vi "数据库读取.vi"(4 "error in (no error)":errorcluster caption="错误输入（无错误）", 6 "Container State":T6 caption="容器状态", 7 "Display State In":T1={"扫描参数"={"+ V"=0.0, "+ Δ V"=0.0, "+ limit I"=0.01, "- V"=0.0, "- Δ V"=0.0, "- limit I"=0.01, "ΔT"=0.0, "NPLC"=0.001}, "保持时间"={"+ V"=0.0, "+ limit I"=0.01, "T"=0.0, "ΔT"=0.0, "NPLC"=0.001}, "功能选择"=enum."扫描", "强制时序"=FALSE, "数据库引用"=refnum} caption="显示状态输入" {"保持时间"."ΔT" format="%#_6ps"; "保持时间"."T" format="%#_6ps"; "保持时间"."NPLC" min=0.001 max=25.0 step=0.001; "保持时间"."+ limit I" min=1e-08 max=3.0 format="%#_6pA"; "保持时间"."+ V" min=-40.0 max=40.0 format="%#_6pV"; "扫描参数"."NPLC" min=0.001 max=25.0 step=0.001; "扫描参数"."- Δ V" min=0.0 max=1.0 format="%#_6pV"; "扫描参数"."+ Δ V" min=0.0 max=1.0 format="%#_6pV"; "扫描参数"."- V" min=-40.0 max=40.0 format="%#_6pV"; "扫描参数"."- limit I" min=1e-08 max=3.0 format="%#_6pA"; "扫描参数"."ΔT" format="%#_6ps"; "扫描参数"."+ limit I" min=1e-08 max=3.0 format="%#_6pA"; "扫描参数"."+ V" min=-40.0 max=40.0 format="%#_6pV"}) -> (0 "error out":errorcluster caption="错误输出", 2 "Value":T5 caption="值", 3 "Display State Out":T1={"扫描参数"={"+ V"=0.0, "+ Δ V"=0.0, "+ limit I"=0.01, "- V"=0.0, "- Δ V"=0.0, "- limit I"=0.01, "ΔT"=0.0, "NPLC"=0.001}, "保持时间"={"+ V"=0.0, "+ limit I"=0.01, "T"=0.0, "ΔT"=0.0, "NPLC"=0.001}, "功能选择"=enum."扫描", "强制时序"=FALSE, "数据库引用"=refnum} caption="显示状态输出" {"保持时间"."ΔT" format="%#_6ps"; "保持时间"."T" format="%#_6ps"; "保持时间"."NPLC" min=0.001 max=25.0 step=0.001; "保持时间"."+ limit I" min=1e-08 max=3.0 format="%#_6pA"; "保持时间"."+ V" min=-40.0 max=40.0 format="%#_6pV"; "扫描参数"."NPLC" min=0.001 max=25.0 step=0.001; "扫描参数"."- Δ V" min=0.0 max=1.0 format="%#_6pV"; "扫描参数"."+ Δ V" min=0.0 max=1.0 format="%#_6pV"; "扫描参数"."- V" min=-40.0 max=40.0 format="%#_6pV"; "扫描参数"."- limit I" min=1e-08 max=3.0 format="%#_6pA"; "扫描参数"."ΔT" format="%#_6ps"; "扫描参数"."+ limit I" min=1e-08 max=3.0 format="%#_6pA"; "扫描参数"."+ V" min=-40.0 max=40.0 format="%#_6pV"})   [LabVIEW 2020, in "功能选择.xctl"]
uses:
  <vilib>/_xctls/Container State.ctl
  <vilib>/_xctls/XControlSupport.lvlib
  <vilib>/addons/database/Connection.llb/Conn ObjectReference.ctl
  <vilib>/addons/database/NI_Database_API.lvlib
panel:
  # "将以下值显示控件替换为所需类型的显示控件。\n不要从连线板中删除该显示控件或其它显示控件。\n不要更改连线板模式。\n值显示控件应始终位于连线板输出端自顶部起第二个接线端。"
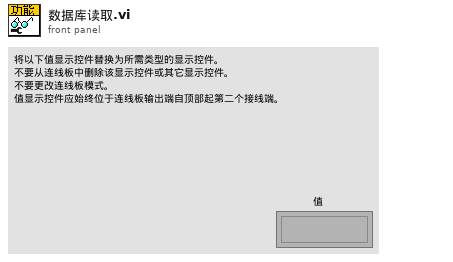
[diagram p1: front panel]
types:
  T1 = typedef "功能选择.xctl/状态.ctl" = cluster{"扫描参数":T2, "保持时间":T3, "功能选择":T4, "强制时序":bool, "数据库引用":T5}
  T2 = typedef "功能选择.xctl/扫描参数.ctl" = cluster{"+ V":dbl, "+ Δ V":dbl, "+ limit I":dbl, "- V":dbl, "- Δ V":dbl, "- limit I":dbl, "ΔT":dbl, "NPLC":dbl}
  T3 = typedef "功能选择.xctl/保持时间.ctl" = cluster{"+ V":dbl, "+ limit I":dbl, "T":dbl, "ΔT":dbl, "NPLC":dbl}
  T4 = typedef "功能选择.xctl/数据.ctl" = enum16{"扫描", "保持时间", "脉冲", "高速脉冲", "任意波形"}
  T5 = typedef "NI_Database_API.lvlib/Conn ObjectReference.ctl" = refnum<k1>
  T6 = typedef "XControlSupport.lvlib/Container State.ctl" = cluster{"Indicator?":bool, "Run Mode?":bool, " Refnum":refnum<vi>}
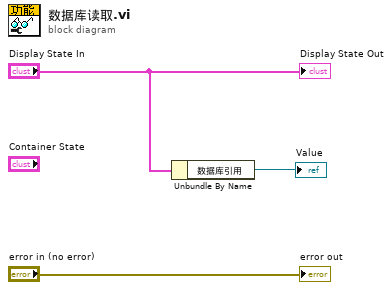
[diagram p0: block diagram]
diagram:
  n1 = Unbundle By Name("Display State In") -> ("数据库引用"=→"Value":T5)
  "error out" <- "error in (no error)"
  "Display State Out" <- "Display State In"
